vi "test_F9P_232-2.vi"() -> ()   [LabVIEW 2019] (continued)
\n$GPGSV,4,4,13,30,01,134,,1*52\r\n$GPGSV,4,1,13,02,65,334,,04,08,037,18,05,48,261,35,06,58,076,34,6*67\r\n$GPGSV,4,2,13,07,06,105,,09,38,057,38,12,18,263,18,13,08,191,,6*6E\r\n$GPGSV,4,3,13,17,19,158,18,19,37,161,,25,11,294,,29,06,323,,6*60\r\n$GPGSV,4,4,13,30,01,134,,6*55\r\n$GLGSV,2,1,06,70,55,030,31,71,68,223,41,72,17,216,29,84,09,133,08,1*74\r\n$GLGSV,2,2,06,85,63,111,30,86,51,337,,1*79\r\n$GLGSV,2,1,06,70,55,030,,71,68,223,28,72,17,216,22,84,09,133,11,3*78\r\n$GLGSV,2,2,06,85,63,111,26,86,51,337,,3*7C\r\n$GAGSV,3,1,09,02,04,288,09,04,68,087,35,09,44,196,26,11,77,034,37,7*76\r\n$GAGSV,3,2,09,12,32,114,26,18,55,286,39,19,17,042,24,25,01,241,,7*79\r\n$GAGSV,3,3,09,36,34,314,24,7*48\r\n$GAGSV,3,1,09,02,04,288,,04,68,087,26,09,44,196,23,11,77,034,30,2*7A\r\n$GAGSV,3,2,09,12,32,114,26,18,55,286,40,19,17,042,31,25,01,241,,2*76\r\n$GAGSV,3,3,09,36,34,314,21,2*48\r\n$GBGSV,4,1,13,04,35,133,,05,09,257,,06,27,182,,07,09,201,,1*7B\r\n$GBGSV,4,2,13,08,65,355,40,09,07,194,,10,16,222,19,11,38,142,25,1*7B\r\n$GBGSV,4,3,13,13,50,314,21,14,77,038,42,28,58,310,30,33,72,237,41,1*79\r\n$GBGSV,4,4,13,34,13,141,,1*45\r\n$GBGSV,4,1,13,04,35,133,,05,09,257,,06,27,182,,07,09,201,,3*79\r\n$GBGSV,4,2,13,08,65,355,32,09,07,194,,10,16,222,20,11,38,142,36,3*74\r\n$GBGSV,4,3,13,13,50,314,,14,77,038,37,28,58,310,,33,72,237,,3*7C\r\n$GBGSV,4,4,13,34,13,141,,3*47\r\n$GNGLL,3723.60513,N,12656.93913,E,064203.00,A,A*77\r\n$GNRMC,064204.00,A,3723.60555,N,12656.93986,E,2.460,62.61,250720,,,A,V*32\r\n$GNVTG,62.61,T,,M,2.460,N,4.556,K,A*12\r\n$GNGGA,064204.00,3723.60555,N,12656.93986,E,1,12,0.62,52.6,M,18.5,M,,*71\r\n$GNGSA,A,3,17,19,06,05,02,12,09,,,,,,1.08,0.62,0.88,1*09\r\n$GNGSA,A,3,85,70,71,72,,,,,,,,,1.08,0.62,0.88,2*06\r\n$GNGSA,A,3,36,19,11,04,09,12,,,,,,,1.08,0.62,0.88,3*0D\r\n$GNGSA,A,3,28,14,13,11,33,08,10,,,,,,1.08,0.62,0.88,4*0D\r\n$GPGSV,4,1,13,02,65,334,46,04,08,037,24,05,48,261,40,06,58,076,41,1*6D\r\n$GPGSV,4,2,13,07,06,105,,09,38,057,44,12,18,263,25,13,08,191,,1*6C\r\n$GPGSV,4,3,13,17,19,158,26,19,37,161,33,25,11,294,26,29,06,323,,1*6E\r\n$GPGSV,4,4,13,30,01,134,,1*52\r\n$GPGSV,4,1,13,02,65,334,,04,08,037,18,05,48,261,30,06,58,076,36,6*60\r\n$GPGSV,4,2,13,07,06,105,,09,38,057,41,12,18,263,16,13,08,191,,6*6E\r\n$GPGSV,4,3,13,17,19,158,18,19,37,161,,25,11,294,,29,06,323,,6*60\r\n$GPGSV,4,4,13,30,01,134,,6*55\r\n$GLGSV,2,1,06,70,55,030,31,71,68,223,39,72,17,216,28,84,09,133,11,1*72\r\n$GLGSV,2,2,06,85,63,111,37,86,51,337,,1*7E\r\n$GLGSV,2,1,06,70,55,030,,71,68,223,23,72,17,216,22,84,09,133,10,3*72\r\n$GLGSV,2,2,06,85,63,111,27,86,51,337,,3*7D\r\n$GAGSV,3,1,09,02,04,288,06,04,68,087,36,09,44,196,31,11,77,034,39,7*72\r\n$GAGSV,3,2,09,12,32,114,25,18,55,286,40,19,17,042,23,25,01,241,,7*73\r\n$GAGSV,3,3,09,36,34,314,22,7*4E\r\n$GAGSV,3,1,09,02,04,288,,04,68,087,28,09,44,196,21,11,77,034,31,2*77\r\n$GAGSV,3,2,09,12,32,114,25,18,55,286,41,19,17,042,28,25,01,241,,2*7C\r\n$GAGSV,3,3,09,36,34,314,17,2*4D\r\n$GBGSV,4,1,13,04,35,133,,05,09,257,,06,27,182,,07,09,201,,1*7B\r\n$GBGSV,4,2,13,08,65,355,38,09,07,194,,10,16,222,19,11,38,142,25,1*74\r\n$GBGSV,4,3,13,13,50,314,20,14,77,038,41,28,58,310,29,33,72,237,38,1*7D\r\n$GBGSV,4,4,13,34,13,141,,1*45\r\n$GBGSV,4,1,13,04,35,133,,05,09,257,,06,27,182,,07,09,201,,3*79\r\n$GBGSV,4,2,13,08,65,355,28,09,07,194,,10,16,222,21,11,38,142,33,3*7B\r\n$GBGSV,4,3,13,13,50,314,,14,77,038,38,28,58,310,,33,72,237,,3*73\r\n$GBGSV,4,4,13,34,13,141,,3*47\r\n$GNGLL,3723.60555,N,12656.93986,E,064204.00,A,A*7E\r\n$GNRMC,064205.00,A,3723.60574,N,12656.94053,E,1.943,68.11,250720,,,A,V*34\r\n$GNVTG,68.11,T,,M,1.943,N,3.599,K,A*14\r\n$GNGGA,064205.00,3723.60574,N,12656.94053,E,1,12,0.64,52.0,M,18.5,M,,*75\r\n$GNGSA,A,3,17,19,06,05,02,12,09,,,,,,1.09,0.64,0.88,1*0E\r\n$GNGSA,A,3,85,70,71,72,,,,,,,,,1.09,0.64,0.88,2*01\r\n$GNGSA,A,3,36,19,11,04,09,12,,,,,,,1.09,0.64,0.88,3*0A\r\n$GNGSA,A,3,28,14,13,11,33,08,10,,,,,,1.09,0.64,0.88,4*0A\r\n$GPGSV,4,1,13,02,65,334,47,04,08,037,22,05,48,261,39,06,58,076,44,1*61\r\n$GPGSV,4,2,13,07,06,105,,09,38,057,42,12,18,263,26,13,08,191,,1*69\r\n$GPGSV,4,3,13,17,19,158,26,19,37,161,38,25,11,294,24,29,06,323,,1*67\r\n$GPGSV,4,4,13,30,01,134,,1*52\r\n$GPGSV,4,1,13,02,65,334,,04,08,037,19,05,48,261,32,06,58,076,31,6*64\r\n$GPGSV,4,2,13,07,06,105,,09,38,057,36,12,18,263,16,13,08,191,,6*6E\r\n$GPGSV,4,3,13,17,19,158,18,19,37,161,,25,11,294,,29,06,323,,6*60\r\n$GPGSV,4,4,13,30,01,134,,6*55\r\n$GLGSV,2,1,06,70,55,030,31,71,68,223,41,72,17,216,28,84,09,133,09,1*74\r\n$GLGSV,2,2,06,85,63,111,30,86,51,337,,1*79\r\n$GLGSV,2,1,06,70,55,030,,71,68,223,24,72,17,216,21,84,09,133,07,3*70\r\n$GLGSV,2,2,06,85,63,111,26,86,51,337,,3*7C\r\n$GAGSV,3,1,09,02,04,288,11,04,68,087,39,09,44,196,25,11,77,034,39,7*7E\r\n$GAGSV,3,2,09,12,32,114,25,18,55,286,40,19,17,042,25,25,01,241,,7*75\r\n$GAGSV,3,3,09,36,34,314,24,7*48\r\n$GAGSV,3,1,09,02,04,288,,04,68,087,31,09,44,196,24,11,77,034,34,2*7F\r\n$GAGSV,3,2,09,12,32,114,26,18,55,286,43,19,17,042,,25,01,241,,2*77\r\n$GAGSV,3,3,09,36,34,314,17,2*4D\r\n$GBGSV,4,1,13,04,35,133,,05,09,257,,06,27,182,,07,09,201,,1*7B\r\n$GBGSV,4,2,13,08,65,355,33,09,07,194,,10,16,222,19,11,38,142,30,1*7B\r\n$GBGSV,4,3,13,13,50,314,20,14,77,038,40,28,58,310,28,33,72,237,39,1*7C\r\n$GBGSV,4,4,13,34,13,141,,1*45\r\n$GBGSV,4,1,13,04,35,133,,05,09,257,,06,27,182,,07,09,201,,3*79\r\n$GBGSV,4,2,13,08,65,355,27,09,07,194,,10,16,222,21,11,38,142,,3*74\r\n$GBGSV,4,3,13,13,50,314,,14,77,038,38,28,58,310,,33,72,237,,3*73\r\n$GBGSV,4,4,13,34,13,141,,3*47\r\n$GNGLL,3723.60574,N,12656.94053,E,064205.00,A,A*7A\r\n$GNRMC,064206.00,A,3723.60590,N,12656.94131,E,2.392,73.75,250720,,,A,V*35\r\n$GNVTG,73.75,T,,M,2.392,N,4.430,K,A*1C\r\n$GNGGA,064206.00,3723.60590,N,12656.94131,E,1,12,0.64,51.8,M,18.5,M,,*72\r\n$GNGSA,A,3,17,19,06,05,02,12,09,,,,,,1.09,0.64,0.88,1*0E\r\n$GNGSA,A,3,85,70,71,72,,,,,,,,,1.09,0.64,0.88,2*01\r\n$GNGSA,A,3,36,19,11,04,09,12,,,,,,,1.09,0.64,0.88,3*0A\r\n$GNGSA,A,3,28,14,13,11,33,08,10,,,,,,1.09,0.64,0.88,4*0A\r\n$GPGSV,4,1,13,02,65,334,36,04,08,037,21,05,48,261,30,06,58,076,32,1*6C\r\n$GPGSV,4,2,13,07,06,105,,09,38,057,39,12,18,263,26,13,08,191,,1*65\r\n$GPGSV,4,3,13,17,19,158,25,19,37,161,30,25,11,294,22,29,06,323,,1*6A\r\n$GPGSV,4,4,13,30,01,134,,1*52\r\n$GPGSV,4,1,13,02,65,334,,04,08,037,18,05,48,261,28,06,58,076,34,6*6B\r\n$GPGSV,4,2,13,07,06,105,,09,38,057,37,12,18,263,16,13,08,191,,6*6F\r\n$GPGSV,4,3,13,17,19,158,16,19,37,161,,25,11,294,,29,06,323,,6*6E\r\n$GPGSV,4,4,13,30,01,134,,6*55\r\n$GLGSV,2,1,06,70,55,030,25,71,68,223,30,72,17,216,26,84,09,133,05,1*75\r\n$GLGSV,2,2,06,85,63,111,32,86,51,337,,1*7B\r\n$GLGSV,2,1,06,70,55,030,,71,68,223,26,72,17,216,20,84,09,133,09,3*7D\r\n$GLGSV,2,2,06,85,63,111,24,86,51,337,,3*7E\r\n$GAGSV,3,1,09,02,04,288,08,04,68,087,37,09,44,196,25,11,77,034,35,7*74\r\n$GAGSV,3,2,09,12,32,114,25,18,55,286,36,19,17,042,25,25,01,241,,7*74\r\n$GAGSV,3,3,09,36,34,314,22,7*4E\r\n$GAGSV,3,1,09,02,04,288,,04,68,087,30,09,44,196,24,11,77,034,30,2*7A\r\n$GAGSV,3,2,09,12,32,114,24,18,55,286,34,19,17,042,,25,01,241,,2*75\r\n$GAGSV,3,3,09,36,34,314,14,2*4E\r\n$GBGSV,4,1,13,04,35,133,,05,09,257,,06,27,182,,07,09,201,,1*7B\r\n$GBGSV,4,2,13,08,65,355,29,09,07,194,,10,16,222,17,11,38,142,29,1*76\r\n$GBGSV,4,3,13,13,50,314,19,14,77,038,38,28,58,310,28,33,72,237,34,1*74\r\n$GBGSV,4,4,13,34,13,141,,1*45\r\n$GBGSV,4,1,13,04,35,133,,05,09,257,,06,27,182,,07,09,201,,3*79\r\n$GBGSV,4,2,13,08,65,355,27,09,07,194,,10,16,222,21,11,38,142,33,3*74\r\n$GBGSV,4,3,13,13,50,314,,14,77,038,37,28,58,310,,33,72,237,,3*7C\r\n$GBGSV,4,4,13,34,13,141,,3*47\r\n$GNGLL,3723.60590,N,12656.94131,E,064206.00,A,A*76\r\n$GNRMC,064207.00,A,3723.60612,N,12656.94217,E,2.505,71.87,250720,,,A,V*3D\r\n$GNVTG,71.87,T,,M,2.505,N,4.640,K,A*1E\r\n$GNGGA,064207.00,3723.60612,N,12656.94217,E,1,12,0.77,51.6,M,18.5,M,,*71\r\n$GNGSA,A,3,17,19,06,05,02,12,09,,,,,,1.19,0.77,0.92,1*06\r\n$GNGSA,A,3,85,70,71,72,,,,,,,,,1.19,0.77,0.92,2*09\r\n$GNGSA,A,3,36,19,11,04,09,12,,,,,,,1.19,0.77,0.92,3*02\r\n$GNGSA,A,3,28,14,13,11,33,08,10,,,,,,1.19,0.77,0.92,4*02\r\n$GPGSV,4,1,13,02,65,334,40,04,08,037,20,05,48,261,30,06,58,076,36,1*68\r\n$GPGSV,4,2,13,07,06,105,,09,38,057,31,12,18,263,24,13,08,191,,1*6F\r\n$GPGSV,4,3,13,17,19,158,25,19,37,161,25,25,11,294,19,29,06,323,,1*66\r\n$GPGSV,4,4,13,30,01,134,,1*52\r\n$GPGSV,4,1,13,02,65,334,,04,08,037,16,05,48,261,29,06,58,076,32,6*62\r\n$GPGSV,4,2,13,07,06,105,,09,38,057,25,12,18,263,15,13,08,191,,6*6F\r\n$GPGSV,4,3,13,17,19,158,17,19,37,161,,25,11,294,,29,06,323,,6*6F\r\n$GPGSV,4,4,13,30,01,134,,6*55\r\n$GLGSV,2,1,06,70,55,030,27,71,68,223,24,72,17,216,22,84,09,133,06,1*75\r\n$GLGSV,2,2,06,85,63,111,22,86,51,337,,1*7A\r\n$GLGSV,2,1,06,70,55,030,,71,68,223,25,72,17,216,18,84,09,133,09,3*75\r\n$GLGSV,2,2,06,85,63,111,23,86,51,337,,3*79\r\n$GAGSV,3,1,09,02,04,288,10,04,68,087,30,09,44,196,26,11,77,034,32,7*7E\r\n$GAGSV,3,2,09,12,32,114,26,18,55,286,33,19,17,042,27,25,01,241,,7*70\r\n$GAGSV,3,3,09,36,34,314,24,7*48\r\n$GAGSV,3,1,09,02,04,288,,04,68,087,34,09,44,196,30,11,77,034,29,2*73\r\n$GAGSV,3,2,09,12,32,114,30,18,55,286,36,19,17,042,,25,01,241,,2*72\r\n$GAGSV,3,3,09,36,34,314,,2*4B\r\n$GBGSV,4,1,13,04,35,133,,05,09,257,,06,27,182,,07,09,201,,1*7B\r\n$GBGSV,4,2,13,08,65,355,29,09,07,194,,10,16,222,16,11,38,142,30,1*7F\r\n$GBGSV,4,3,13,13,50,314,17,14,77,038,31,28,58,310,20,33,72,237,32,1*7D\r\n$GBGSV,4,4,13,34,13,141,,1*45\r\n$GBGSV,4,1,13,04,35,133,,05,09,257,,06,27,182,,07,09,201,,3*79\r\n$GBGSV,4,2,13,08,65,355,25,09,07,194,,10,16,222,19,11,38,142,31,3*7F\r\n$GBGSV,4,3,13,13,50,314,,14,77,038,34,28,58,310,,33,72,237,,3*7F\r\n$GBGSV,4,4,13,34,13,141,,3*47\r\n$GNGLL,3723.60612,N,12656.94217,E,064207.00,A,A*79\r\n$GNRMC,064208.00,A,3723.60625,N,12656.94303,E,2.465,77.32,250720,,,A,V*3D\r\n$GNVTG,77.32,T,,M,2.465,N,4.566,K,A*16\r\n$GNGGA,064208.00,3723.60625,N,12656.94303,E,1,12,0.68,51.4,M,18.5,M,,*72\r\n$GNGSA,A,3,17,19,06,05,02,12,09,,,,,,1.12,0.68,0.90,1*01\r\n$GNGSA,A,3,85,70,71,72,,,,,,,,,1.12,0.68,0.90,2*0E\r\n$GNGSA,A,3,36,19,11,04,09,12,,,,,,,1.12,0.68,0.90,3*05\r\n$GNGSA,A,3,28,14,13,11,33,08,10,,,,,,1.12,0.68,0.90,4*05\r\n$GPGSV,4,1,13,02,65,334,36,04,08,037,21,05,48,261,31,06,58,076,31,1*6E\r\n$GPGSV,4,2,13,07,06,105,,09,38,057,27,12,18,263,23,13,08,191,,1*6F\r\n$GPGSV,4,3,13,17,19,158,25,19,37,161,26,25,11,294,17,29,06,323,,1*6B\r\n$GPGSV,4,4,13,30,01,134,,1*52\r\n$GPGSV,4,1,13,02,65,334,,04,08,037,15,05,48,261,28,06,58,076,32,6*60\r\n$GPGSV,4,2,13,07,06,105,,09,38,057,35,12,18,263,15,13,08,191,,6*6E\r\n$GPGSV,4,3,13,17,19,158,17,19,37,161,,25,11,294,,29,06,323,,6*6F\r\n$GPGSV,4,4,13,30,01,134,,6*55\r\n$GLGSV,2,1,06,70,55,030,27,71,68,223,23,72,17,216,15,84,09,133,06,1*76\r\n$GLGSV,2,2,06,85,63,111,22,86,51,337,,1*7A\r\n$GLGSV,2,1,06,70,55,030,,71,68,223,24,72,17,216,17,84,09,133,12,3*71\r\n$GLGSV,2,2,06,85,63,111,23,86,51,337,,3*79\r\n$GAGSV,3,1,09,02,04,288,08,04,68,087,26,09,44,196,25,11,77,034,32,7*73\r\n$GAGSV,3,2,09,12,32,114,25,18,55,286,30,19,17,042,19,25,01,241,,7*7D\r\n$GAGSV,3,3,09,36,34,314,22,7*4E\r\n$GAGSV,3,1,09,02,04,288,,04,68,087,30,09,44,196,21,11,77,034,28,2*76\r\n$GAGSV,3,2,09,12,32,114,22,18,55,286,40,19,17,042,25,25,01,241,,2*77\r\n$GAGSV,3,3,09,36,34,314,,2*4B\r\n$GBGSV,4,1,13,04,35,133,,05,09,257,,06,27,182,,07,09,201,,1*7B\r\n$GBGSV,4,2,13,08,65,355,29,09,07,194,,10,16,222,13,11,38,142,24,1*7F\r\n$GBGSV,4,3,13,13,50,314,17,14,77,038,32,28,58,310,21,33,72,237,26,1*7A\r\n$GBGSV,4,4,13,34,13,141,,1*45\r\n$GBGSV,4,1,13,04,35,133,,05,09,257,,06,27,182,,07,09,201,,3*79\r\n$GBGSV,4,2,13,08,65,355,25,09,07,194,,10,16,222,18,11,38,142,37,3*78\r\n$GBGSV,4,3,13,13,50,314,,14,77,038,33,28,58,310,,33,72,237,,3*78\r\n$GBGSV,4,4,13,34,13,141,,3*47\r\n$GNGLL,3723.60625,N,12656.94303,E,064208.00,A,A*76\r\n$GNRMC,064209.00,A,3723.60642,N,12656.94370,E,1.816,78.39,250720,,,A,V*36\r\n$GNVTG,78.39,T,,M,1.816,N,3.364,K,A*1A\r\n$GNGGA,064209.00,3723.60642,N,12656.94370,E,1,12,0.65,51.5,M,18.5,M,,*7A\r\n$GNGSA,A,3,17,19,06,05,02,12,09,,,,,,1.11,0.65,0.90,1*0F\r\n$GNGSA,A,3,85,70,71,72,,,,,,,,,1.11,0.65,0.90,2*00\r\n$GNGSA,A,3,36,19,11,04,09,12,,,,,,,1.11,0.65,0.90,3*0B\r\n$GNGSA,A,3,28,14,13,11,33,08,10,,,,,,1.11,0.65,0.90,4*0B\r\n$GPGSV,4,1,13,02,65,334,35,04,08,037,19,05,48,261,27,06,58,076,36,1*66\r\n$GPGSV,4,2,13,07,06,105,,09,38,057,34,12,18,263,22,13,08,191,,1*6C\r\n$GPGSV,4,3,13,17,19,158,24,19,37,161,26,25,11,294,,29,06,323,,1*6C\r\n$GPGSV,4,4,13,30,01,134,,1*52\r\n$GPGSV,4,1,13,02,65,334,,04,08,037,15,05,48,261,19,06,58,076,29,6*68\r\n$GPGSV,4,2,13,07,06,105,,09,38,057,25,12,18,263,15,13,08,191,,6*6F\r\n$GPGSV,4,3,13,17,19,158,16,19,37,161,,25,11,294,,29,06,323,,6*6E\r\n$GPGSV,4,4,13,30,01,134,,6*55\r\n$GLGSV,2,1,06,70,55,030,26,71,68,223,23,72,17,216,13,84,09,133,07,1*70\r\n$GLGSV,2,2,06,85,63,111,23,86,51,337,,1*7B\r\n$GLGSV,2,1,06,70,55,030,,71,68,223,22,72,17,216,17,84,09,133,13,3*76\r\n$GLGSV,2,2,06,85,63,111,25,86,51,337,,3*7F\r\n$GAGSV,3,1,09,02,04,288,09,04,68,087,37,09,44,196,23,11,77,034,36,7*70\r\n$GAGSV,3,2,09,12,32,114,23,18,55,286,34,19,17,042,20,25,01,241,,7*75\r\n$GAGSV,3,3,09,36,34,314,19,7*46\r\n$GAGSV,3,1,09,02,04,288,,04,68,087,30,09,44,196,21,11,77,034,27,2*79\r\n$GAGSV,3,2,09,12,32,114,22,18,55,286,29,19,17,042,24,25,01,241,,2*79\r\n$GAGSV,3,3,09,36,34,314,,2*4B\r\n$GBGSV,4,1,13,04,35,133,,05,09,257,,06,27,182,,07,09,201,,1*7B\r\n$GBGSV,4,2,13,08,65,355,20,09,07,194,,10,16,222,,11,38,142,31,1*70\r\n$GBGSV,4,3,13,13,50,314,13,14,77,038,38,28,58,310,23,33,72,237,31,1*70\r\n$GBGSV,4,4,13,34,13,141,,1*45\r\n$GBGSV,4,1,13,04,35,133,,05,09,257,,06,27,182,,07,09,201,,3*79\r\n$GBGSV,4,2,13,08,65,355,26,09,07,194,,10,16,222,17,11,38,142,29,3*7B\r\n$GBGSV,4,3,13,13,50,314,23,14,77,038,34,28,58,310,,33,72,237,,3*7E\r\n$GBGSV,4,4,13,34,13,141,,3*47\r\n$GNGLL,3723.60642,N,12656.94370,E,064209.00,A,A*72\r\n$GNRMC,064210.00,A,3723.60659,N,12656.94423,E,1.498,76.34,250720,,,A,V*3C\r\n$GNVTG,76.34,T,,M,1.498,N,2.774,K,A*17\r\n$GNGGA,064210.00,3723.60659,N,12656.94423,E,1,12,0.71,51.2,M,18.5,M,,*7B\r\n$GNGSA,A,3,17,19,06,05,02,12,09,,,,,,1.14,0.71,0.90,1*0F\r\n$GNGSA,A,3,85,70,71,72,,,,,,,,,1.14,0.71,0.90,2*00\r\n$GNGSA,A,3,36,19,11,04,09,12,,,,,,,1.14,0.71,0.90,3*0B\r\n$GNGSA,A,3,28,14,13,11,33,08,10,,,,,,1.14,0.71,0.90,4*0B\r\n$GPGSV,4,1,13,02,65,334,39,04,08,037,21,05,48,261,38,06,58,076,45,1*6B\r\n$GPGSV,4,2,13,07,06,105,,09,38,057,34,12,18,263,23,13,08,191,,1*6D\r\n$GPGSV,4,3,13,17,19,158,22,19,37,161,26,25,11,294,,29,07,323,,1*6B\r\n$GPGSV,4,4,13,30,01,134,,1*52\r\n$GPGSV,4,1,13,02,65,334,,04,08,037,17,05,48,261,36,06,58,076,29,6*67\r\n$GPGSV,4,2,13,07,06,105,,09,38,057,32,12,18,263,16,13,08,191,,6*6A\r\n$GPGSV,4,3,13,17,19,158,16,19,37,161,,25,11,294,,29,07,323,,6*6F\r\n$GPGSV,4,4,13,30,01,134,,6*55\r\n$GLGSV,2,1,06,70,55,030,26,71,68,223,39,72,17,216,12,84,09,133,09,1*74\r\n$GLGSV,2,2,06,85,63,111,26,86,51,337,,1*7E\r\n$GLGSV,2,1,06,70,55,030,,71,68,223,30,72,17,216,17,84,09,133,15,3*73\r\n$GLGSV,2,2,06,85,63,111,26,86,51,337,,3*7C\r\n$GAGSV,3,1,09,02,04,288,09,04,68,087,44,09,44,196,24,11,77,034,39,7*7C\r\n$GAGSV,3,2,09,12,32,114,24,18,55,286,46,19,17,042,22,25,01,241,,7*75\r\n$GAGSV,3,3,09,36,34,314,20,7*4C\r\n$GAGSV,3,1,09,02,04,288,,04,68,087,38,09,44,196,29,11,77,034,35,2*7A\r\n$GAGSV,3,2,09,12,32,114,22,18,55,286,44,19,17,042,30,25,01,241,,2*77\r\n$GAGSV,3,3,09,36,34,314,25,2*4C\r\n$GBGSV,4,1,13,04,35,133,,05,09,257,,06,27,182,,07,09,201,,1*7B\r\n$GBGSV,4,2,13,08,65,355,20,09,07,194,,10,16,222,,11,38,142,38,1*79\r\n$GBGSV,4,3,13,13,50,314,15,14,77,038,42,28,58,310,23,33,72,237,40,1*7D\r\n$GBGSV,4,4,13,34,13,141,,1*45\r\n$GBGSV,4,1,13,04,35,133,,05,09,257,,06,27,182,,07,09,201,,3*79\r\n$GBGSV,4,2,13,08,65,355,26,09,07,194,,10,16,222,17,11,38,142,29,3*7B\r\n$GBGSV,4,3,13,13,50,314,23,14,77,038,36,28,58,310,,33,72,237,,3*7C\r\n$GBGSV,4,4,13,34,13,141,,3*47\r\n$GNGLL,3723.60659,N,12656.94423,E,064210.00,A,A*71\r\n$GNRMC,064211.00,A,3723.60698,N,12656.94492,E,2.508,71.88,250720,,,A,V*31\r\n$GNVTG,71.88,T,,M,2.508,N,4.645,K,A*19\r\n$GNGGA,064211.00,3723.60698,N,12656.94492,E,1,12,0.68,51.2,M,18.5,M,,*75\r\n$GNGSA,A,3,17,19,06,05,02,12,09,,,,,,1.13,0.68,0.90,1*00\r\n$GNGSA,A,3,85,70,71,72,,,,,,,,,1.13,0.68,0.90,2*0F\r\n$GNGSA,A,3,36,19,11,04,09,12,,,,,,,1.13,0.68,0.90,3*04\r\n$GNGSA,A,3,28,14,13,11,33,08,10,,,,,,1.13,0.68,0.90,4*04\r\n$GPGSV,4,1,13,02,65,334,35,04,08,037,21,05,48,261,36,06,58,076,47,1*6B\r\n$GPGSV,4,2,13,07,06,105,,09,38,057,35,12,18,263,23,13,08,191,,1*6C\r\n$GPGSV,4,3,13,17,19,158,22,19,37,161,26,25,11,294,19,29,07,323,19,1*6B\r\n$GPGSV,4,4,13,30,01,134,,1*52\r\n$GPGSV,4,1,13,02,65,334,,04,08,037,18,05,48,261,38,06,58,076,31,6*6F\r\n$GPGSV,4,2,13,07,06,105,,09,38,057,32,12,18,263,16,13,08,191,,6*6A\r\n$GPGSV,4,3,13,17,19,158,17,19,37,161,,25,11,294,24,29,07,323,,6*68\r\n$GPGSV,4,4,13,30,01,134,,6*55\r\n$GLGSV,2,1,06,70,55,030,28,71,68,223,41,72,17,216,23,84,09,133,10,1*7F\r\n$GLGSV,2,2,06,85,63,111,37,86,51,337,,1*7E\r\n$GLGSV,2,1,06,70,55,030,,71,68,223,37,72,17,216,20,84,09,133,13,3*76\r\n$GLGSV,2,2,06,85,63,111,26,86,51,337,,3*7C\r\n$GAGSV,3,1,09,02,04,288,07,04,68,087,41,09,44,196,33,11,77,034,38,7*70\r\n$GAGSV,3,2,09,12,32,114,32,18,55,286,46,19,17,042,24,25,01,241,,7*74\r\n$GAGSV,3,3,09,36,34,314,20,7*4C\r\n$GAGSV,3,1,09,02,04,288,,04,68,087,36,09,44,196,33,11,77,034,31,2*7B\r\n$GAGSV,3,2,09,12,32,114,21,18,55,286,43,19,17,042,22,25,01,241,,2*70\r\n$GAGSV,3,3,09,36,34,314,24,2*4D\r\n$GBGSV,4,1,13,04,35,133,,05,09,257,,06,27,182,,07,09,201,,1*7B\r\n$GBGSV,4,2,13,08,65,355,29,09,07,194,,10,16,222,,11,38,142,29,1*70\r\n$GBGSV,4,3,13,13,50,314,18,14,77,038,41,28,58,310,31,33,72,237,42,1*72\r\n$GBGSV,4,4,13,34,13,141,,1*45\r\n$GBGSV,4,1,13,04,35,133,,05,09,257,,06,27,182,,07,09,201,,3*79\r\n$GBGSV,4,2,13,08,65,355,27,09,07,194,,10,16,222,19,11,38,142,29,3*74\r\n$GBGSV,4,3,13,13,50,314,22,14,77,038,35,28,58,310,,33,72,237,,3*7E\r\n$GBGSV,4,4,13,34,13,141,,3*47\r\n$GNGLL,3723.60698,N,12656.94492,E,064211.00,A,A*77\r\n$GNRMC,064212.00,A,3723.60756,N,12656.94562,E,2.762,58.93,250720,,,A,V*30\r\n$GNVTG,58.93,T,,M,2.762,N,5.116,K,A*16\r\n$GNGGA,064212.00,3723.60756,N,12656.94562,E,1,12,0.71,50.6,M,18.5,M,,*76\r\n$GNGSA,A,3,17,19,06,05,02,12,09,,,,,,1.14,0.71,0.90,1*0F\r\n$GNGSA,A,3,85,70,71,72,,,,,,,,,1.14,0.71,0.90,2*00\r\n$GNGSA,A,3,36,19,11,04,09,12,,,,,,,1.14,0.71,0.90,3*0B\r\n$GNGSA,A,3,28,14,13,11,33,08,10,,,,,,1.14,0.71,0.90,4*0B\r\n$GPGSV,4,1,13,02,65,334,35,04,08,037,28,05,48,261,44,06,58,076,45,1*65\r\n$GPGSV,4,2,13,07,06,105,,09,38,057,37,12,18,263,28,13,08,191,,1*65\r\n$GPGSV,4,3,13,17,19,158,30,19,37,161,25,25,11,294,22,29,07,323,15,1*6F\r\n$GPGSV,4,4,13,30,01,134,,1*52\r\n$GPGSV,4,1,13,02,65,334,,04,08,037,18,05,48,261,37,06,58,076,31,6*60\r\n$GPGSV,4,2,13,07,06,105,,09,38,057,33,12,18,263,19,13,08,191,,6*64\r\n$GPGSV,4,3,13,17,19,158,19,19,37,161,,25,11,294,20,29,07,323,,6*62\r\n$GPGSV,4,4,13,30,01,134,,6*55\r\n$GLGSV,2,1,06,70,55,030,29,71,68,223,42,72,17,216,29,84,09,133,15,1*72\r\n$GLGSV,2,2,06,85,63,111,37,86,51,337,,1*7E\r\n$GLGSV,2,1,06,70,55,030,,71,68,223,34,72,17,216,20,84,09,133,14,3*72\r\n$GLGSV,2,2,06,85,63,111,26,86,51,337,,3*7C\r\n$GAGSV,3,1,09,02,04,288,08,04,68,087,41,09,44,196,30,11,77,034,41,7*72\r\n$GAGSV,3,2,09,12,32,114,25,18,55,286,45,19,17,042,25,25,01,241,,7*70\r\n$GAGSV,3,3,09,36,34,314,19,7*46\r\n$GAGSV,3,1,09,02,04,288,,04,68,087,36,09,44,196,23,11,77,034,34,2*7F\r\n$GAGSV,3,2,09,12,32,114,21,18,55,286,42,19,17,042,23,25,01,241,,2*70\r\n$GAGSV,3,3,09,36,34,314,22,2*4B\r\n$GBGSV,4,1,13,04,35,133,,05,09,257,,06,27,182,,07,09,201,,1*7B\r\n$GBGSV,4,2,13,08,65,355,32,09,07,194,,10,16,222,,11,38,142,32,1*70\r\n$GBGSV,4,3,13,13,50,314,19,14,77,038,44,28,58,310,27,33,72,237,43,1*70\r\n$GBGSV,4,4,13,34,13,141,,1*45\r\n$GBGSV,4,1,13,04,35,133,,05,09,257,,06,27,182,,07,09,201,,3*79\r\n$GBGSV,4,2,13,08,65,355,26,09,07,194,,10,16,222,19,11,38,142,27,3*7B\r\n$GBGSV,4,3,13,13,50,314,20,14,77,038,26,28,58,310,,33,72,237,,3*7E\r\n$GBGSV,4,4,13,34,13,141,,3*47\r\n$GNGLL,3723.60756,N,12656.94562,E,064212.00,A,A*79\r\n$GNRMC,064213.00,A,3723.60796,N,12656.94619,E,1.932,58.97,250720,,,A,V*3E\r\n$GNVTG,58.97,T,,M,1.932,
